vi "Read user events.vi"(11 "Generic Optimization in":refnum<class "Generic Optimization.lvclass">) -> (2 "user events":T1, 3 "Generic Optimization out":refnum<class "Generic Optimization.lvclass">)   [LabVIEW 2016]
uses:
  Generic Optimization.lvclass
  C:/Users/Administrator/Desktop/LabVIEW EMS/SCADA Sub Abstract Actor/SCADA Sub Abstract/SCADA Sub Abstract.lvclass
  C:/Users/Administrator/Desktop/LabVIEW EMS/EMS Generic Actor/EMS Generic/EMS Generic.lvclass
  C:/Program Files (x86)/National Instruments/LabVIEW 2016/vi.lib/ActorFramework/Actor/Actor.lvclass
  EMS Generic Actor/EMS Generic/Controls/EMS Generic User Events.ctl
  EMS Generic Actor/EMS Generic/EMS Generic.lvclass
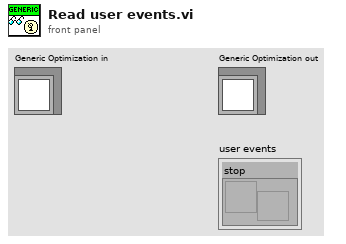
[diagram p1: front panel]
types:
  T1 = typedef "EMS Generic Actor.lvlib/EMS Generic.lvclass/EMS Generic User Events.ctl" = cluster{"stop":refnum<user-event>}
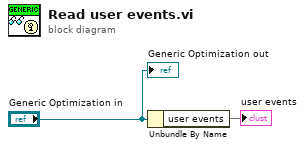
[diagram p0: block diagram]
diagram:
  n1 = Unbundle By Name("Generic Optimization in") -> ("user events"=→"user events")
  "Generic Optimization out" <- "Generic Optimization in"
